vi "Output_ON_DSP.vi"(8 "error in":errorcluster caption="에러 입력", 11 "VISA":refnum<visa-resource-name>) -> (0 "error out":errorcluster caption="에러 출력", 3 "VISA  Out":refnum<visa-resource-name>)   [LabVIEW 2019]
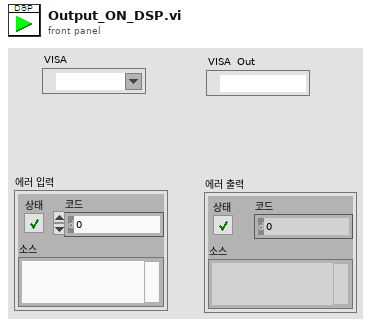
[diagram p1: front panel]
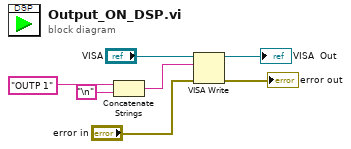
[diagram p0: block diagram]
diagram:
  n1 = Concatenate Strings("OUTP 1", "\n") -> (w6:string)
  n2 = VISA Write(VISA resource name="VISA", write buffer=w6, error in (no error)="error in") -> (VISA resource name out=→"VISA  Out":refnum<visa-resource-name>, error out=→"error out":errorcluster)  [unwired: 1 out]
